vi "Get or Create Template.vi"(8 "error in (no error)":errorcluster, 10 "Base Folder":path) -> (0 "error out":errorcluster, 3 "Template Clone Ref":refnum<vi>)   [LabVIEW 2019, in "GOOP Probe.lvlib"]
uses:
  GOOP Probe.lvlib
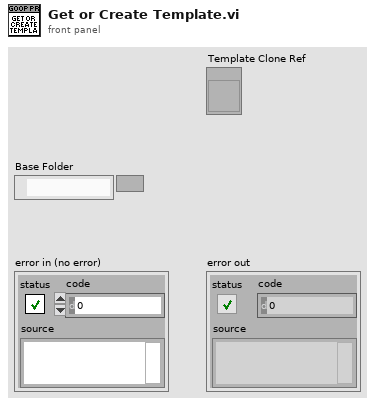
[diagram p1: front panel]
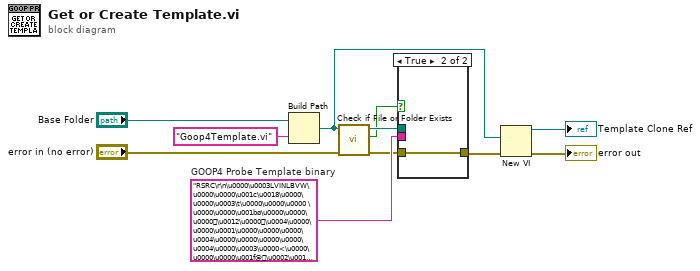
[diagram p0: block diagram]
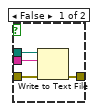
[diagram p2: hidden frame]
diagram:
  w9 = "RSRC\r\n\u0000\u0003LVINLBVW\u0000\u0000\u001c\u0018\u0000\u0000\u0003\t\u0000\u0000\u0000 \u0000\u0000\u001bø\u0000\u0000\u0000\u0012\u0000\u0004\u0000\u0000\u0001\u0000\u0000\u0000\u0004\u0000\u0000\u0000\u0000\u0004\u0000\u0003\u0000<\u0000\u0000\u0000\u001f@\u0002\u0010\u0000\u0000\u0000\u0001\u0000\u0001\u0000\u0002ÿÿÿÿ\u0000\u0000\u0000\u0000\u0000\u0000\u0000\u0000\u0000\u0000\u0000\u0000VK`ËÿçFÜEÂ\u0013\u001dëÊ\u0000\u0000\u0000\f\u0000\u0000\u0000\u0010\u0000\u0000\u0000\u0000Ï_\u0016t4³pNAL\u0012°aÔ\u001dÙ\u0000²\u0004é\tìøB~\u0000\u0000\u0010\u0000\u0000\u0000\u0000\u0000OGñå§ZqF°K\u0011nô\u0016\u0000\u0000\u0000\u0010j\u001dþáñÎi\u001b\u001e1\u0012Yê#\"\u0000\u0000\u0000\f\u0012\u0000$\u0000\u0000\u000412.0\u0000\u0000\u0000\u0000\u0002\u0000\u0001\u0000\u0000\u0000\u0000\u0000 \u0000\u0001LVIN\u0010Goop4Template.vi\u0000\u0000\u0000\u0000\u0000\u0000\u0000\u0000\u0003\u0000\u0000\u00000Ô\u001dÙ\u0000²\u0004é\tìøB~å\u001dFú\tÔ\nvV\u000e©øÄÖÂüáÕ¾qÕwJ\u0012Âí^c\u0000\u0000\u0000ÿÿÿÿ\u0000\u0000\u0001\u0000\u0000\u0001\u0000\u0000\u0001\u0000\u0000\u0001\u0000\u0000\u0001\u0000\u0000\u00011\u0011JR1J\\QJPq1\u0011\u0000\u0000\u0001\u0000\u0000\u0001\u0000\u0000\u0001\u0000\u0000\u0001\u0000\u0000\u0001\u0000\u0000\u0001\u0000\u0000\u0001qáJRr\\ÁJRIá\u0000\u0000\u0001\u0000\u0000\u0001\u0000\u0000\u0001\u0000\u0000\u0001\u0000\u0000\u0001\u0000\u0000\u0001\u0000\u0000\u0001ÿÿÿÿ\u0000\u0000\u0002\u0000ÿÿÿÿÿÿÿÿÿÿÿÿÿÿÿÿøøøøøøøÿÿøÿøøøøøÿøøÿøøÿ..."  # GOOP4 Probe Template binary
  n1 = Build Path(base path="Base Folder", name or relative path="Goop4Template.vi") -> (appended path=w4:path)
  n2 = call <vilib>:"Check if File or Folder Exists.vi"("error in (no error)"="error in (no error)", "path"=w4) -> ("error out"=w8:errorcluster, "file or folder exists?"=w6:bool, "dup path"=w7:path)  [unwired: 7 in]
  n3 = case shown="True" w6 {
    tunnel: w7 -> [w12 _]
    tunnel: w9 -> [w15 _]
    tunnel: w8 -> [w14 w16]
    tunnel: [w13 w16] -> w5
    frame False {
      n4 = Write to Text File(file (use dialog)=w12, text=w15, error in=w14) -> (error out=w13:errorcluster)  [unwired: 1 in, 2 out]
    }
    frame True {
    }
  }
  n5 = New VI(8:w5, 10:w4) -> (0:→"error out":errorcluster, 3:→"Template Clone Ref":refnum<vi>)  [unwired: 5 in]
